vi "LANGUAGE.vi"() -> ()   [LabVIEW 2015]
uses:
  Controls/HID Data.ctl
  <vilib>/userdefined/High Color/IMAQdx.ctl
  <vilib>/vision/Image Controls.llb/IMAQ Image.ctl
  Controls/HID State.ctl
  Controls/FGV_Options.ctl
panel:
  in  "TXT_004":string
  in  "Language":u16(ring) items=["English", "Español", "Português"]
  in  "BOOL_004":bool
  in  "BOOL_003":bool
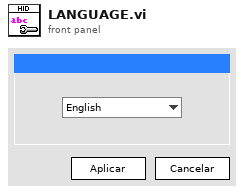
[diagram p1: front panel]
types:
  T1 = typedef "FGV_Options.ctl" = enum16{"Read from File", "Write to File", "Get", "Set"}
  T2 = typedef "HID Data.ctl" = cluster{"IMAQdx Session":T3, "Resampled Image":T4, "Low Level Grab":T4, "X Resolution":i32, "Y Resolution":i32, "Image Threshold":u8, "Reset Value":i32, "FIFO Timer":u16, "Row Timer":u32, "Memory Writer Timer":u8, "Color":enum16{"Green", "Blue", "Red", "White", "Pink", "Yellow", "Turquoise", "Black"}, "Top":bool[][], "Bottom":bool[][], "Timeout (ms)":i32, "Menu Tag":string, "Color Background":enum16{"Green", "Blue", "Red", "White", "Pink", "Yellow", "Turquoise", "Black"}, "FPGA VI Reference":refnum<k20>, "Next Steps":T5[], "Turn off LED Matrix":bool, "FPGA Alias":string, "FPGA Bitfile":path, "Localized Texts":cluster{"Status Text":cluster{"Status Text Table":string[], "Status Text Index":i32}, "Controls":cluster{"Control Text Table":string[], "Control Text Index":i32}, "Titles":cluster{"Titles Text Table":string[], "Titles Text Index":i32}}, "Language":u16}
  T3 = typedef "IMAQdx.ctl" = refnum<k21>
  T4 = typedef "IMAQ Image.ctl" = refnum<image>
  T5 = typedef "HID State.ctl" = enum16{"Initialize", "Set FPGA Parametes", "Set Camera Parameters", "Set LED Matrix Parameters", "Initialize FPGA Interface", "Initialize Camera", "Start FPGA VI", "Start Camera", "Wait for Event", "Update UI", "Acquire", "Process Image", "Get Boolean Arrays", "Send to FPGA", "Menu Pop-Up", "Menu Actions", "Handle Errors", "Close Camera", "Close FPGA", "Stop", "Exit"}
  T6 = cluster{"Status Text":cluster{"Status Text Table":string[], "Status Text Index":i32}, "Controls":cluster{"Control Text Table":string[], "Control Text Index":i32}, "Titles":cluster{"Titles Text Table":string[], "Titles Text Index":i32}}
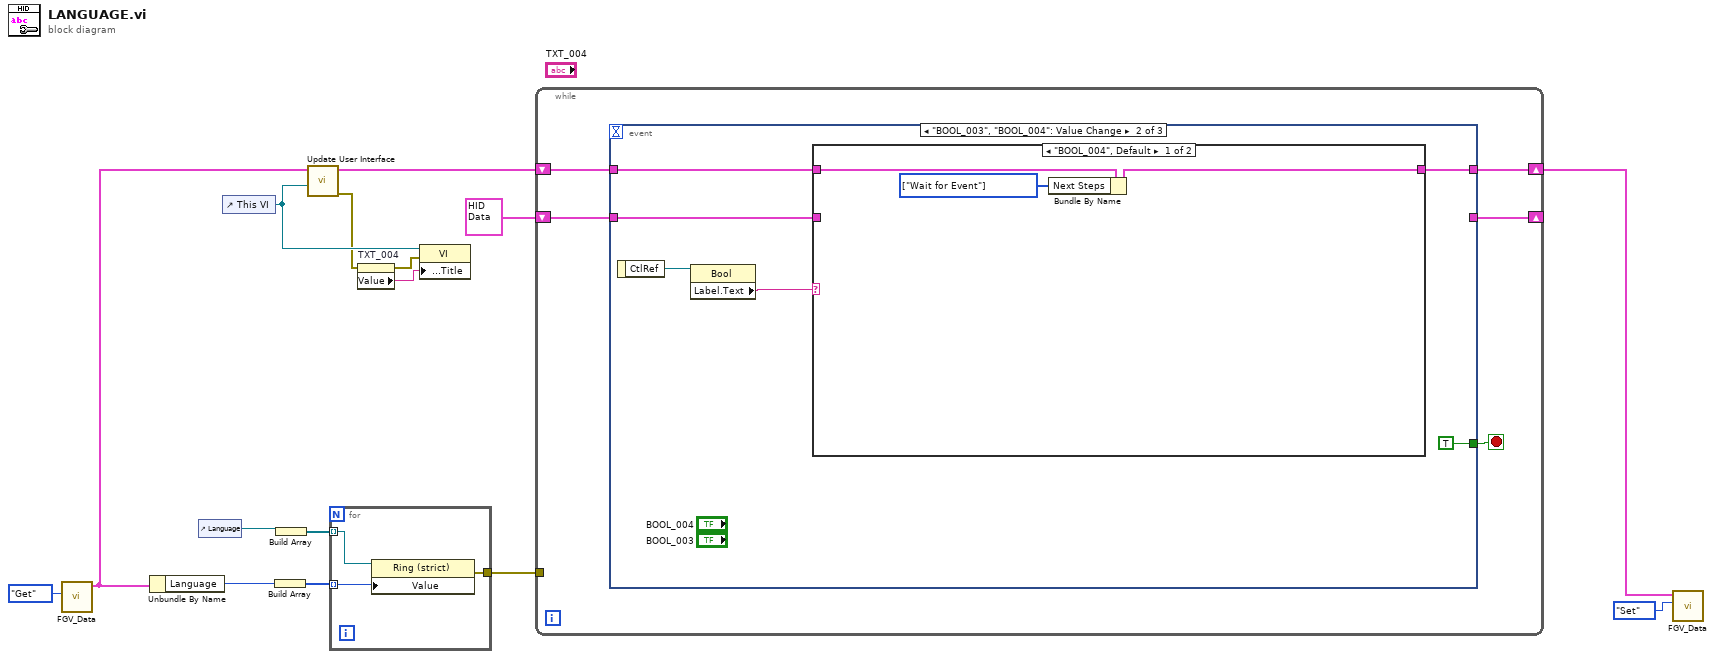
[diagram p0: block diagram]
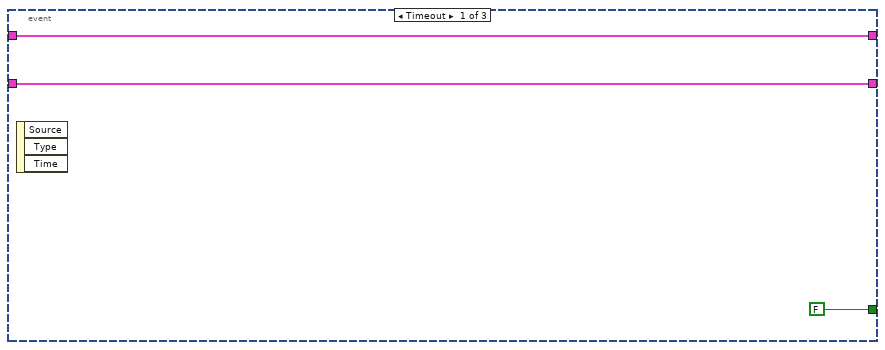
[diagram p2: hidden frame]
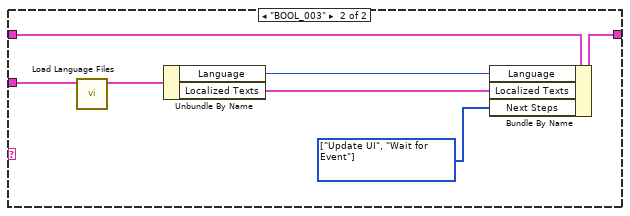
[diagram p3: hidden frame]
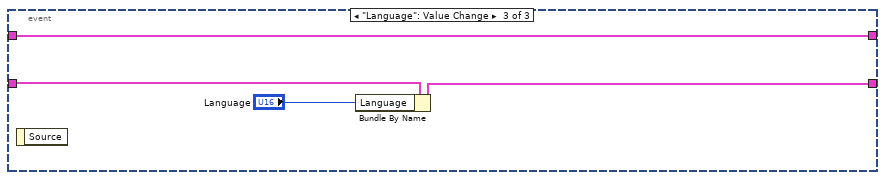
[diagram p4: hidden frame]
diagram:
  n1 = call "FGV_Data.vi"("Option"=FGV_Options."Get") -> ("Data Out"=w8:T2)  [unwired: 9 in, 1 out]
  n2 = Unbundle By Name(w8) -> ("Language"=w13:u16)
  n3 = control-ref of="Language"() -> (w10:refnum<vi>)
  n4 = control-ref of="This VI"() -> (w4:refnum<vi>)
  n5 = Build Array(w13) -> (w14:u16[])
  n6 = Build Array(w10) -> (w12:refnum<vi>[])
  n7 = call "Update User Interface.vi"("VI Refnum"=w4, "Data In"=w8) -> ("error out"=w2:errorcluster, "Data Out"=w5:T2)  [unwired: 8 in]
  n8 = for {
    tunnel: w12 -> [w16] mode=indexing
    tunnel: w14 -> [w18] mode=indexing
    tunnel: [w17] -> w11
    n9 = property class="Ring (strict)"(reference=w16, "Value"=w18) -> (error out=w17:errorcluster)  [unwired: 1 in, 1 out]
  }
  n10 = property on="TXT_004" class="Str"(error in=w2) -> (error out=w3:errorcluster, "Value"=w1:string)  [unwired: 1 in, 1 out]
  n11 = property class="VI"(reference=w4, error in=w3, "Front Panel.Title"=w1) -> ()  [unwired: 2 out]
  n12 = while {
    shift-right: [w23] -> w9
    shift-left: w5 -> [w22]
    shift-right: [w19] -> _
    shift-left: T2 {"IMAQdx Session"="", "Resampled Image"=refnum, "Low Level Grab"=refnum, "X Resolution"=0, "Y Resolution"=0, "Image Threshold"=0, "Reset Value"=0, "FIFO Timer"=0, "Row Timer"=0, "Memory Writer Timer"=0, "Color"=enum."Red", "Top"=array32x96[3072 elements], "Bottom"=array32x96[3072 elements], "Timeout (ms)"=0, "Menu Tag"="", "Color Background"=enum."White", "FPGA VI Reference"=refnum, "Next Steps"=[], "Turn off LED Matrix"=FALSE, "FPGA Alias"="", "FPGA Bitfile"=path "", "Localized Texts"={"Status Text"={"Status Text Table"=[], "Status Text Index"=0}, "Controls"={"Control Text Table"=[], "Control Text Index"=0}, "Titles"={"Titles Text Table"=[], "Titles Text Index"=0}}, "Language"=0} ("Data In TMP") -> [w20]
    tunnel: w11 -> [_]
    stop <- w21 stop-if-true
    n13 = event shown="[1] \"BOOL_003\", \"BOOL_004\": Value Change" {
      selector: _ -> [_ _ _]
      dyn-events: _ -> [_ _ _]
      timeout: _ -> [_ _ _]
      tunnel: [w26 w29 w46] -> w23
      tunnel: w22 -> [w26 w30 w46]
      tunnel: [FALSE TRUE _] -> w21
      tunnel: w20 -> [w24 w27 w44]
      tunnel: [w24 _ w45] -> w19
      event Timeout {
        n14 = event-data() -> ()  [unwired: 1 in, 3 out]
      }
      event "BOOL_003", "BOOL_004": Value Change {
        n15 = event-data() -> ("CtlRef"=w31:refnum<vi>)  [unwired: 1 in]
        n16 = property class="Bool"(reference=w31) -> ("Label.Text"=w28:string)  [unwired: 1 in, 2 out]
        n17 = case shown="\"BOOL_004\", Default" w28 {
          tunnel: w30 -> [w35 w42]
          tunnel: [w34 w41] -> w29
          tunnel: w27 -> [_ w39]
          frame "BOOL_004", Default {
            w33 = T5[] [enum."Wait for Event"] items=["Initialize", "Set FPGA Parametes", "Set Camera Parameters", "Set LED Matrix Parameters", "Initialize FPGA Interface", "Initialize Camera", "Start FPGA VI", "Start Camera", "Wait for Event", "Update UI", "Acquire", "Process Image", "Get Boolean Arrays", "Send to FPGA", "Menu Pop-Up", "Menu Actions", "Handle Errors", "Close Camera", "Close FPGA", "Stop", "Exit"] ("Next Steps")
            n18 = Bundle By Name(cluster=w35, "Next Steps"=w33) -> (w34:T2)
          }
          frame "BOOL_003" {
            w40 = T5[] [enum."Update UI", enum."Wait for Event"] items=["Initialize", "Set FPGA Parametes", "Set Camera Parameters", "Set LED Matrix Parameters", "Initialize FPGA Interface", "Initialize Camera", "Start FPGA VI", "Start Camera", "Wait for Event", "Update UI", "Acquire", "Process Image", "Get Boolean Arrays", "Send to FPGA", "Menu Pop-Up", "Menu Actions", "Handle Errors", "Close Camera", "Close FPGA", "Stop", "Exit"] ("Next Steps")
            n19 = call "Load Language Files.vi"("Data In"=w39) -> ("Data Out"=w38:T2)  [unwired: 10 in]
            n20 = Unbundle By Name(w38) -> ("Language"=w37:u16, "Localized Texts"=w36:T6)
            n21 = Bundle By Name(cluster=w42, "Language"=w37, "Localized Texts"=w36, "Next Steps"=w40) -> (w41:T2)
          }
        }
      }
      event "Language": Value Change {
        n22 = event-data() -> ()  [unwired: 1 in, 1 out]
        n23 = Bundle By Name(cluster=w44, "Language"="Language") -> (w45:T2)
      }
    }
  }
  n24 = call "FGV_Data.vi"("Option"=FGV_Options."Set", "Data In"=w9) -> ()  [unwired: 8 in, 2 out]
